vi "Search for NI Package.vi"(10 "software package ID":string="ni-daqmx-labview-support", 11 "Host Resources":T1) -> (2 "Is package installed?":bool)   [LabVIEW 2021, in "Acquisition.lvlib"]
doc: "Search the NI Software list in 'Host Resources' for 'software package ID'. If present, return TRUE for 'Is package installed?'"
uses:
  Acquisition.lvlib
  Host Resources.ctl
  Host Software Package.ctl
  Host IO Resource.ctl
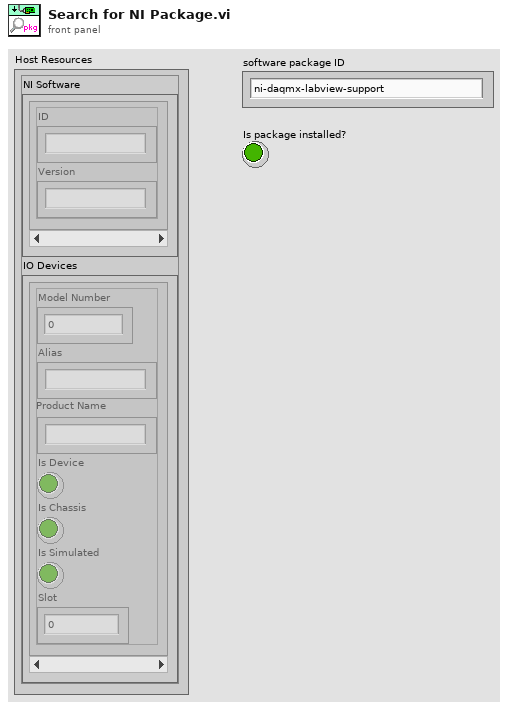
[diagram p1: front panel]
types:
  T1 = typedef "Acquisition.lvlib/Host Resources.ctl" = cluster{"NI Software":T2[], "IO Devices":T3[]}
  T2 = typedef "Acquisition.lvlib/Host Software Package.ctl" = cluster{"ID":string, "Version":string}
  T3 = typedef "Acquisition.lvlib/Host IO Resource.ctl" = cluster{"Model Number":u32, "Alias":string, "Product Name":string, "Is Device":bool, "Is Chassis":bool, "Is Simulated":bool, "Slot":i32}
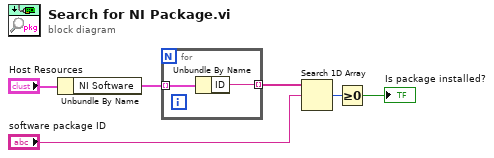
[diagram p0: block diagram]
diagram:
  n1 = Unbundle By Name("Host Resources") -> ("NI Software"=w1:T2[])
  n2 = for {
    tunnel: w1 -> [w8] mode=indexing
    tunnel: [w7] -> w3 mode=indexing
    n3 = Unbundle By Name(w8) -> ("ID"=w7:string)
  }
  n4 = Search 1D Array(1D array=w3, element="software package ID") -> (index of element=w6:i32)  [unwired: 1 in]
  n5 = Greater Or Equal To 0?(x=w6) -> (x >= 0?=→"Is package installed?":bool)
